vi "Get Comma Separated Values_Headers.vi"(8 "Error In":errorcluster, 11 "Output String":string) -> (0 "Error In 2":errorcluster, 3 "Array":string[](array[string]))   [LabVIEW 2017, in "Data Operations.lvlib"]
uses:
  Data Operations.lvlib
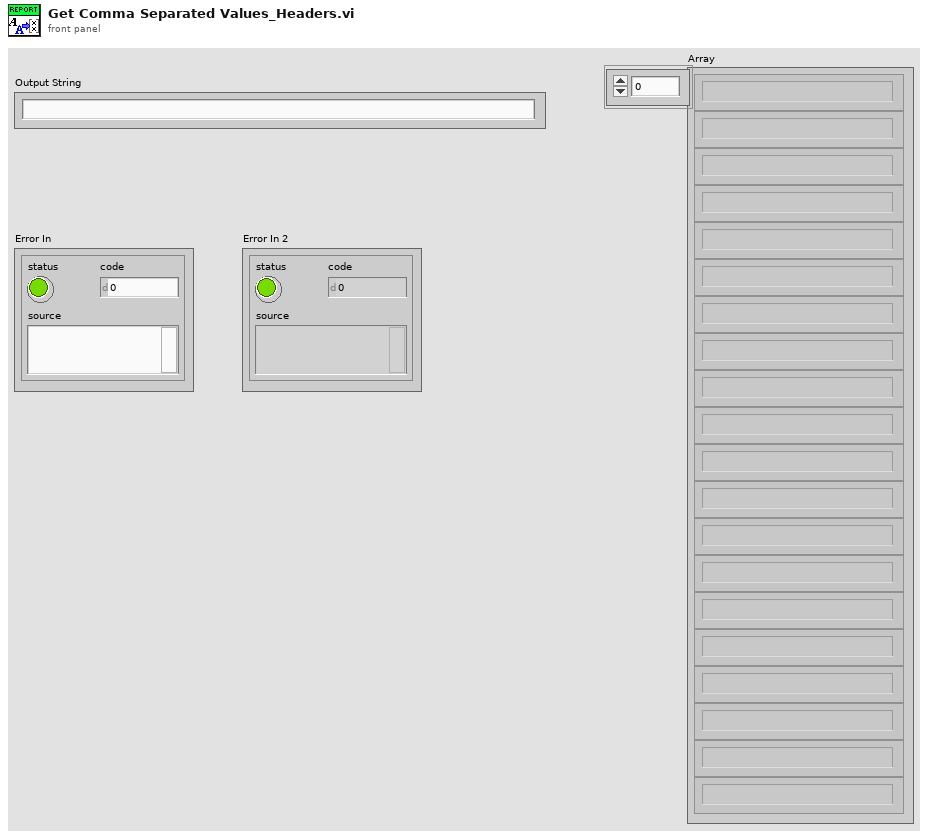
[diagram p1: front panel]
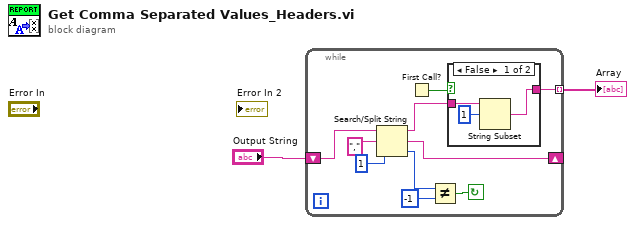
[diagram p0: block diagram]
diagram:
  n1 = while {
    tunnel: [w6] -> w2 mode=indexing
    shift-right: [w10] -> _
    shift-left: "Output String" -> [w12]
    stop <- w3 continue-if-true
    n2 = Search/Split String(string=w12, search string/char (-)=",", offset (0)=1) -> (substring before match=w8:string, match + rest of string=w10:string, offset of match=w5:i32)
    n3 = First Call?() -> (First Call?: T/F=w7:bool)
    n4 = Not Equal?(x=w5, y=-1) -> (x != y?=w3:bool)
    n5 = case shown="False" w7 {
      tunnel: w8 -> [w15 w16]
      tunnel: [w13 w16] -> w6
      frame False {
        n6 = String Subset(string=w15, offset (0)=1) -> (substring=w13:string)  [unwired: 1 in]
      }
      frame True {
      }
    }
  }
  "Array" <- w2
